vi "MinerToUpperCase.vi"(1 "expected":string="af533d87a1b7513b82fe9058af16d86792c98532") -> (0 "UpperExpected":string="af533d87a1b7513b82fe9058af16d86792c98532")   [LabVIEW 2014]
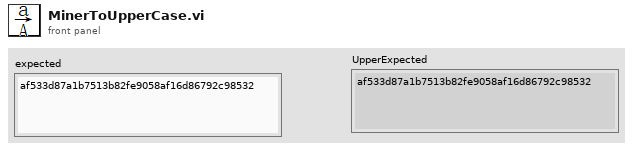
[diagram p1: front panel]
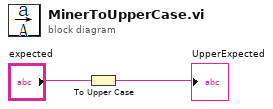
[diagram p0: block diagram]
diagram:
  n1 = To Upper Case(1:"expected") -> (0:→"UpperExpected":string)
